vi "Subiva Creation.vi"(0 "X":dbl, 1 "Y":dbl) -> (2 "(X^2) + (y^2)":dbl, 3 "x > y?":bool, 4 "x < y?":bool, 5 "x = y?":bool)   [LabVIEW 2022 SP3]
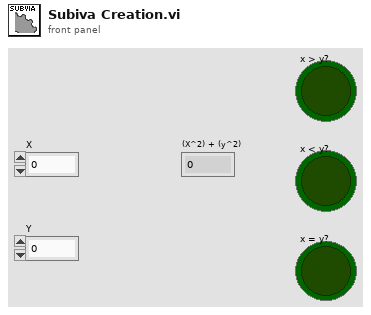
[diagram p1: front panel]
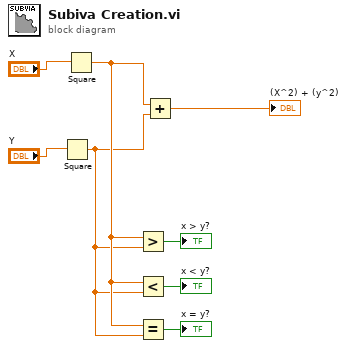
[diagram p0: block diagram]
diagram:
  n1 = Square(x="Y") -> (x^2=w4:dbl)
  n2 = Square(x="X") -> (x^2=w5:dbl)
  n3 = Greater?(x=w5, y=w4) -> (0:→"x > y?":bool)
  n4 = Less?(x=w5, y=w4) -> (x < y?=→"x < y?":bool)
  n5 = Equal?(x=w5, y=w4) -> (x = y?=→"x = y?":bool)
  n6 = Add(x=w5, y=w4) -> (x+y=→"(X^2) + (y^2)":dbl)
